vi "mark_BV.vi"(1 "输入":i8[](array[numeric]), 2 "n":dbl=3.0) -> (0 "输出":i8[](array[numeric]))   [LabVIEW 2018]
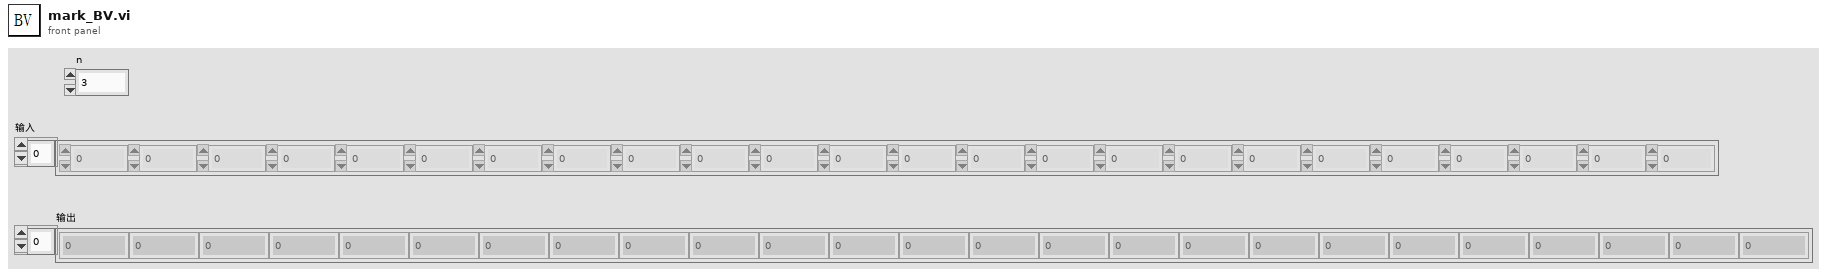
[diagram p1: front panel]
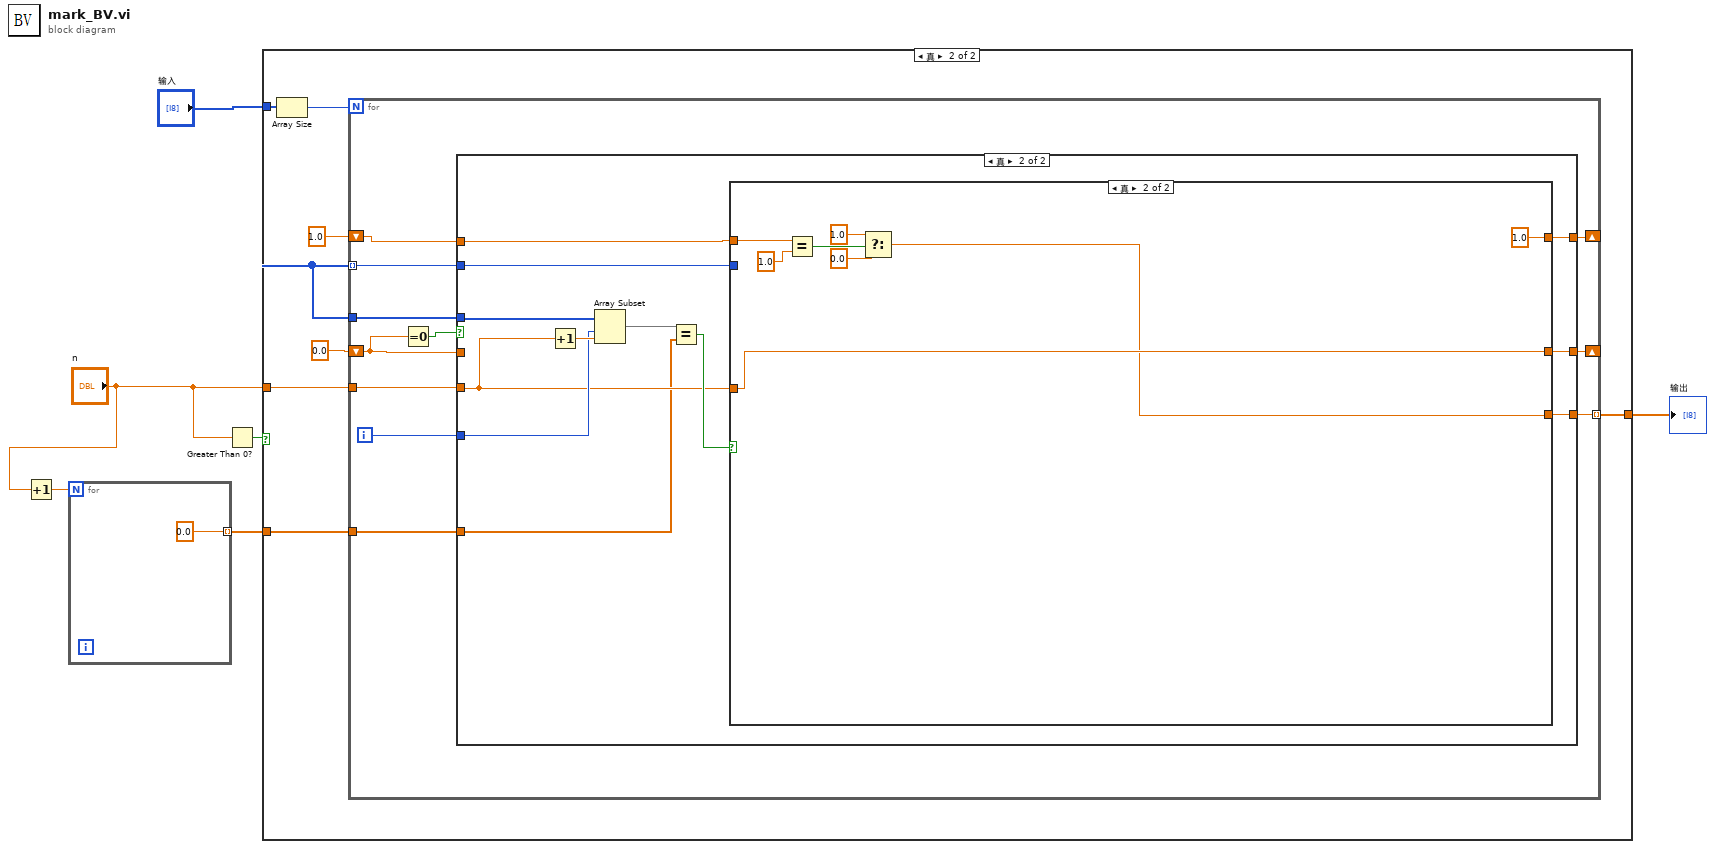
[diagram p0: block diagram]
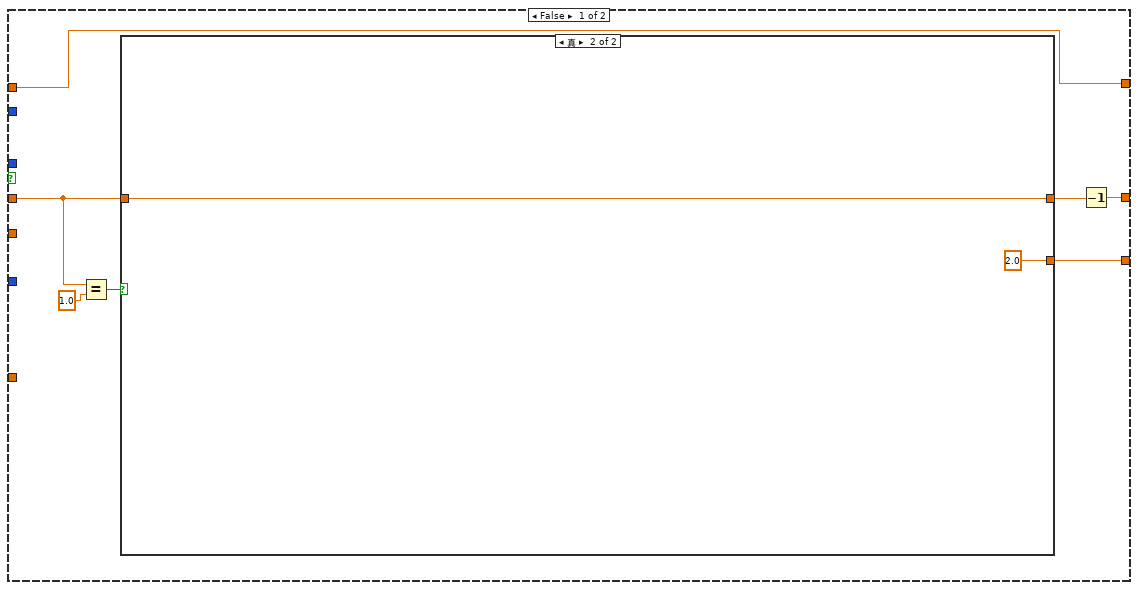
[diagram p3: hidden frame]
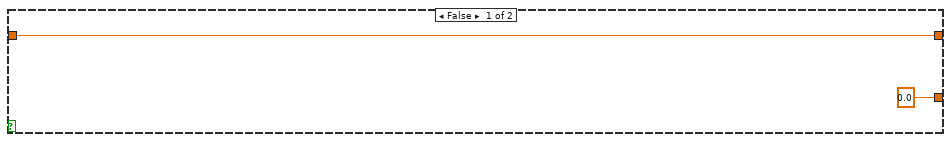
[diagram p4: hidden frame]
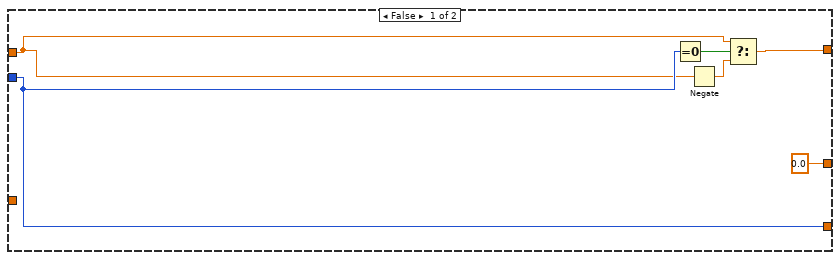
[diagram p5: hidden frame]
diagram:
  n1 = Increment(x="n") -> (x+1=w3:dbl)
  n2 = for {
    N: w3 -> [_]
    tunnel: [0.0] -> w1 mode=indexing
  }
  n3 = Greater Than 0?(x="n") -> (x > 0?=w4:bool)
  n4 = case shown="真" w4 {
    tunnel: "输入" -> [w8 w14]
    tunnel: [w8 w12] -> w5
    tunnel: "n" -> [_ w10]
    tunnel: w1 -> [_ w9]
    frame False {
    }
    frame True {
      n5 = Array Size(array=w14) -> (size(s)=w15:i32)
      n6 = for {
        N: w15 -> [_]
        tunnel: w14 -> [w20] mode=indexing
        tunnel: w14 -> [w26]
        shift-right: [w22] -> _
        shift-left: 0.0 -> [w23]
        tunnel: [w21] -> w12 mode=indexing
        shift-right: [w18] -> _
        shift-left: 1.0 -> [w19]
        tunnel: w10 -> [w17]
        tunnel: w9 -> [w16]
        i -> [w25]
        n7 = Equal To 0?(x=w23) -> (x = 0?=w24:bool)
        n8 = case shown="真" w24 {
          tunnel: w26 -> [_ w49]
          tunnel: w17 -> [_ w41]
          tunnel: w25 -> [_ w46]
          tunnel: w23 -> [w30 _]
          tunnel: [w33 w44] -> w22
          tunnel: [w28 w42] -> w21
          tunnel: w20 -> [_ w43]
          tunnel: w19 -> [w27 w40]
          tunnel: [w27 w39] -> w18
          tunnel: w16 -> [_ w38]
          frame False {
            n9 = Equal?(x=w30, y=1.0) -> (x = y?=w31:bool)
            n10 = case shown="真" w31 {
              tunnel: w30 -> [w35 w37]
              tunnel: [w35 w37] -> w32
              tunnel: [0.0 2.0] -> w28
              frame False {
              }
              frame True {
              }
            }
            n11 = Decrement(x=w32) -> (x-1=w33:dbl)
          }
          frame True {
            n12 = Increment(x=w41) -> (x+1=w48:dbl)
            n13 = Array Subset(array=w49, index=w46, length=w48) -> (w47:i8[])
            n14 = Equal?(x=w47, y=w38) -> (x = y?=w45:bool)
            n15 = case shown="真" w45 {
              tunnel: [0.0 w63] -> w44
              tunnel: w43 -> [w53 _]
              tunnel: [w53 w56] -> w42
              tunnel: w41 -> [_ w63]
              tunnel: w40 -> [w51 w61]
              tunnel: [w50 1.0] -> w39
              frame False {
                n16 = Equal To 0?(x=w53) -> (x = 0?=w54:bool)
                n17 = Negate(x=w51) -> (-x=w52:dbl)
                n18 = Select(t=w51, s=w54, f=w52) -> (s? t:f=w50:dbl)
              }
              frame True {
                n19 = Equal?(x=w61, y=1.0) -> (x = y?=w59:bool)
                n20 = Select(t=1.0, s=w59, f=0.0) -> (s? t:f=w56:dbl)
              }
            }
          }
        }
      }
    }
  }
  "输出" <- w5
